vi "Acqusition & Generation (with Snapshot 3) test.vi"() -> ()   [LabVIEW 2014]
uses:
  <vilib>/Platform/TimedLoop/XDataNode/timing_clust.ctl
  <vilib>/Platform/TimedLoop/XDataNode/nitl_modes.ctl
  <vilib>/Platform/TimedLoop/XDataNode/wakeup.ctl
  <vilib>/rvi/Emulation/niFpgaSctlEmulationGetInTimedLoop.vi
  <vilib>/rvi/Emulation/niFpgaEmulationReportErrorSimple.vi
  <vilib>/rvi/Emulation/niFpgaGetClockAttributes.vi
  <vilib>/rvi/Emulation/niFpgaCriticalErrorInLSC.vi
  <vilib>/rvi/Emulation/niFpgaEmulationIsFPGAContextNoSignature.vi
  <vilib>/rvi/errors/niFpgaSetErrorForExecOnDevCompSimple.vi
  <vilib>/rvi/eio/common/nirviEmuReportErrorAndStop.vi
  <vilib>/rvi/DataTransferAndStorage/Container/Common/niFpgaContainerGetUniqueNameForEmu.vi
  <vilib>/rvi/FIFO/Fifo_Resource/nirvififoEmulationSetSize.vi
  <vilib>/rvi/FIFO/Fifo_Resource/nirviFifoEmulationQueueMgr.vi
  <instcachedir>/0/nirviFifoEmulationQueueMgr_E5CAEC123FF24DC58D834DCA3CDAA9B5.lvgen/nirviFifoEmulationQueueMgr_E5CAEC123FF24DC58D834DCA3CDAA9B5_010.vi
  <vilib>/rvi/FIFO/Fifo_Resource/nirvififoEmulationDetermineInputValidOut.vi
  <vilib>/rvi/FIFO/Fifo_Resource/nirvififoEmulationCreateLock.vi
  <vilib>/rvi/Emulation/niFpgaProcessEmulError.vi
  <vilib>/rvi/FIFO/Fifo_Resource/nirvififoEmulationObtainLock.vi
  <vilib>/rvi/FIFO/Fifo_Resource/nirvififoEmulationReleaseLock.vi
  <vilib>/rvi/occurrence/nirviWaitOnOccurrenceBase.vi
  <vilib>/rvi/errors/nirviReportUnexpectedCaseInternalError.vi
  <vilib>/rvi/errors/nirviReportUnexpectedCaseInternalError (U32).vi
  <vilib>/rvi/Memory/Memory_Emulation/nirvimemoryFastEmulation.vi
  <vilib>/rvi/Memory/Memory_Emulation/nirvimemoryEmulation.vi
  <vilib>/rvi/interface/RandomDataEmulation/niFpgaRandomDataHandleErrors.vi
  <vilib>/rvi/eio/common/nirviEmuTemplateMethod_errors.vi
  <vilib>/Platform/TimedLoop/XDataNode/XDataNode.xnode
  <vilib>/rvi/DataTransferAndStorage/Container/XNode/niFpgaContainer.xnode
  <vilib>/rvi/FIFO/Fifo_Resource/nirvififoEmulationWrite.vi
  <vilib>/rvi/interface/RandomDataEmulation/nirviRandomDataFpgaReadWriteTemplate.vi
  <vilib>/rvi/FIFO/Fifo_Resource/nirvififoEmulationRead.vi
  <vilib>/eio/EIOMethodNode/EIOMethodNode.xnode
  <vilib>/Platform/TimedLoop/XDataNode/XDNodeRunTimeDep.lvlib
panel:
  in  "Snapshot":bool
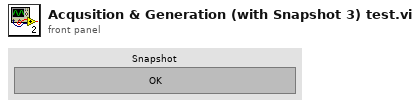
[diagram p1: front panel]
types:
  T1 = typedef "XDNodeRunTimeDep.lvlib/timing_clust.ctl" = cluster{"Expected End [f-1]":u64, "Actual End [f-1]":u64, "Finished Late? [f-1]":bool, "Expected End [i-1]":u64, "Actual End [i-1]":u64, "Finished Late? [i-1]":bool, "Expected Start [i]":u64, "Actual Start [i]":u64, "Expected Start [f]":u64, "Actual Start [f]":u64, "Source Name":string, "Structure Name":string, "Period":i64, "Deadline":i64, "Offset":i64, "Start":i64, "Priority":i32, "Timeout":i32, "Mode":T2, "Wakeup Reason":T3, "Error":errorcluster, "Source Type":string, "Secondary Source Type":string, "Global End Time":u64, "Global Start Time":u64, "Frame Duration":u64, "Iteration Duration":u64, "Assigned CPU":i32, "I/O Scan Engine Mode":u32}
  T2 = typedef "XDNodeRunTimeDep.lvlib/nitl_modes.ctl" = enum32{"No Change", "Process missed periods, maintain original phase", "Discard missed periods, maintain original phase", "Process missed periods, ignore original phase", "Discard missed periods, ignore original phase"}
  T3 = typedef "XDNodeRunTimeDep.lvlib/wakeup.ctl" = enum32{"Normal", "Aborted", "Asynchronous wakeup", "Timing source error", "Timed loop error", "Timeout"}
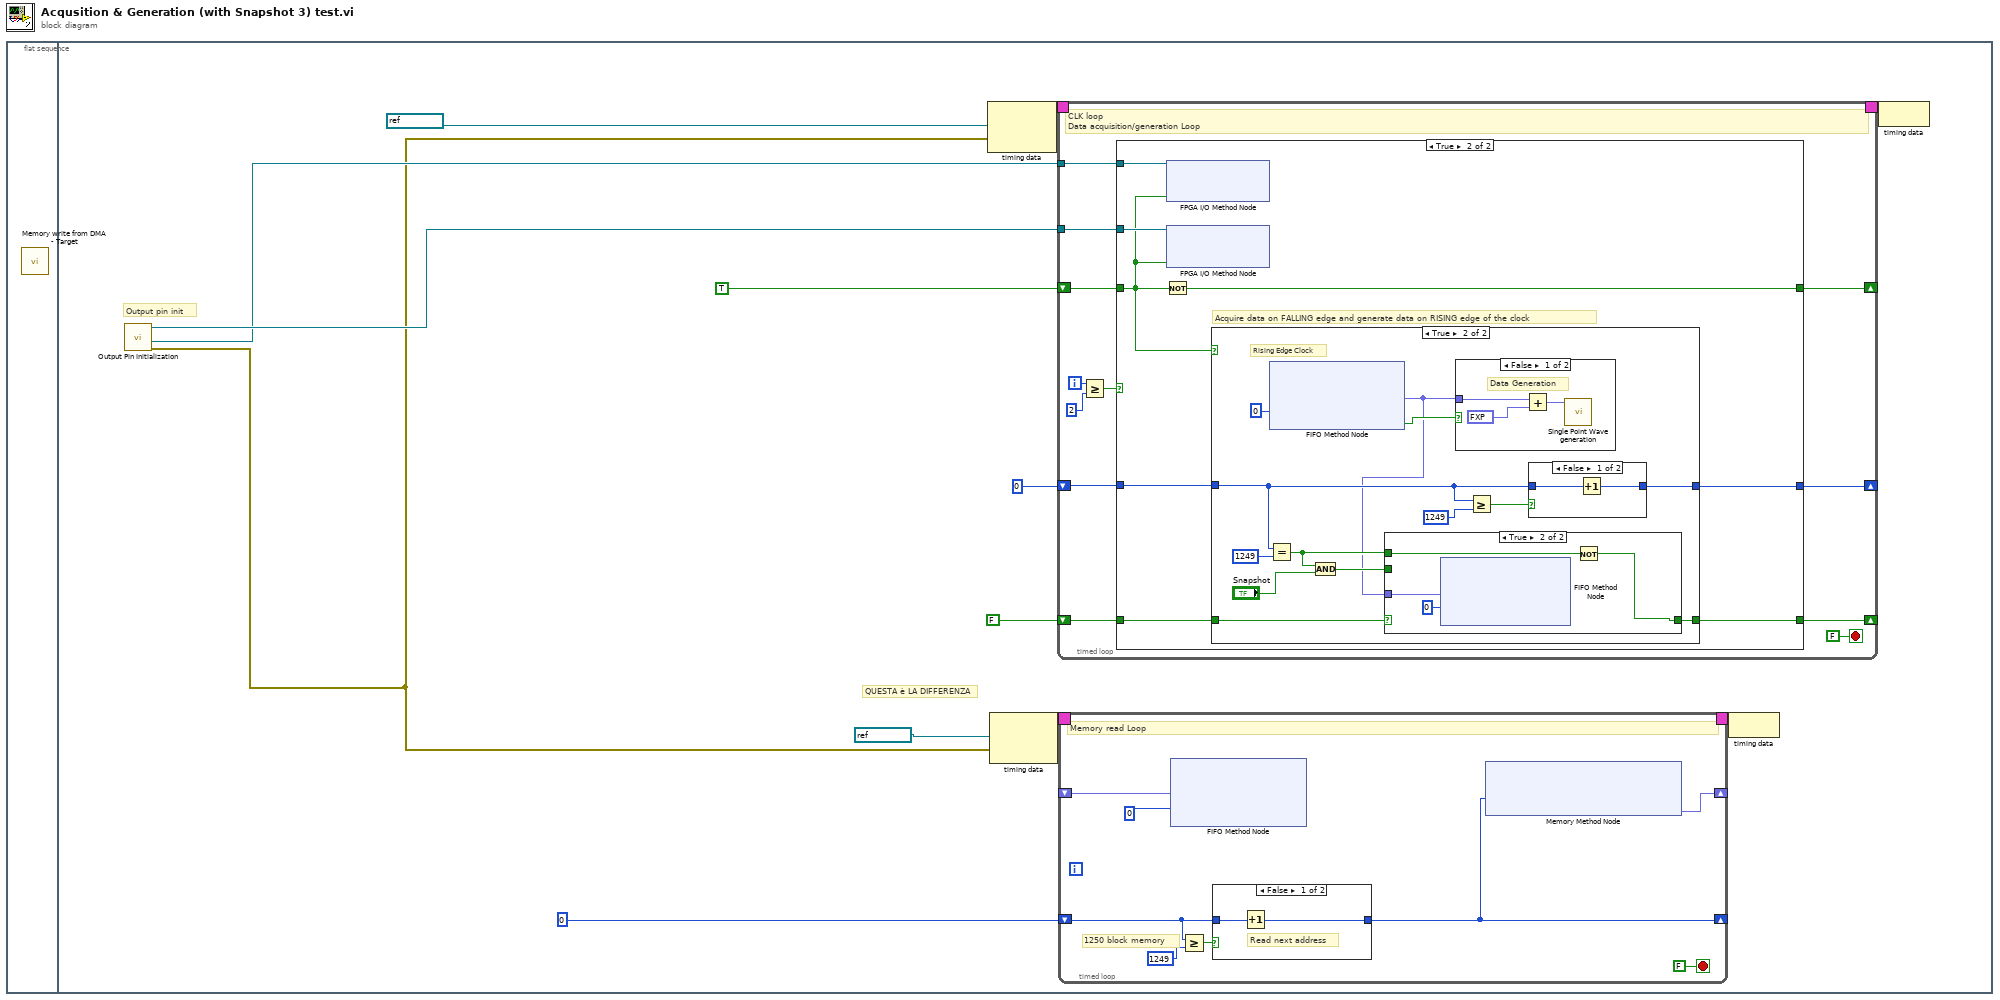
[diagram p0: block diagram]
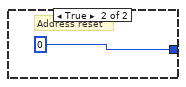
[diagram p2: hidden frame]
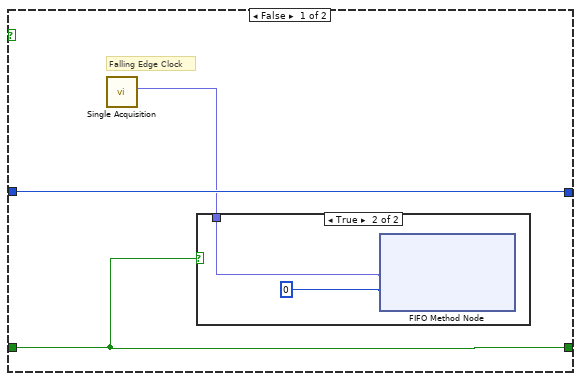
[diagram p4: hidden frame]
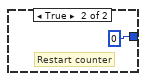
[diagram p8: hidden frame]
diagram:
  n1 = flat-sequence {
    frame #0 {
      n2 = call "Memory write from DMA - Target.vi"() -> ()  [unwired: 12 in]
    }
    frame #1 {
      # "QUESTA è LA DIFFERENZA"
      # "Output pin init"
      n3 = call "Output Pin Initialization.vi"() -> ("error out"=w3:errorcluster, "I/O Out Clock DAC (pin16)"=w4:refnum<k21>, "I/O Out Clock ADC (pin17)"=w5:refnum<k21>)  [unwired: 8 in]
      n4 = node-c288(refnum<k21> "100MHz" ("Source Name"), w3) -> (w13:T1)
      n5 = node-c288(refnum<k21> "100MHz" ("Source Name"), w3) -> (w11:T1)
      n6 = timed-loop {
        timing: w13 -> [_]
        timing-out: [_] -> w12
        shift-right: [w41] -> _
        shift-left: TRUE -> [w39]
        tunnel: w4 -> [w43]
        tunnel: w5 -> [w40]
        shift-right: [w38] -> _
        shift-left: i16 0 -> [w37]
        shift-right: [w35] -> _
        shift-left: FALSE -> [w36]
        i -> [w34]
        stop <- FALSE stop-if-true
        # "CLK loop\nData acquisition/generation Loop"
        n7 = Greater Or Equal?(x=w34, y=2) -> (x >= y?=w32:bool)
        n8 = case shown="True" w32 {
          tunnel: w43 -> [_ w54]
          tunnel: [w46 w53] -> w41
          tunnel: w40 -> [_ w52]
          tunnel: w39 -> [w46 w51]
          tunnel: [w45 w50] -> w38
          tunnel: w37 -> [w45 w49]
          tunnel: w36 -> [w44 w48]
          tunnel: [w44 w47] -> w35
          frame False {
          }
          frame True {
            # "Acquire data on FALLING edge and generate data on RISING edge of the clock"
            n9 = Not(x=w51) -> (.not. x?=w53:bool)
            n10 = xnode "FPGA I/O Method Node"("FPGA I/O In"=w54, "Data"=w51) -> ()  [unwired: 1 out]
            n11 = xnode "FPGA I/O Method Node"("FPGA I/O In"=w52, "Data"=w51) -> ()  [unwired: 1 out]
            n12 = case shown="True" w51 {
              tunnel: [w57 w70] -> w50
              tunnel: w49 -> [w57 w64]
              tunnel: w48 -> [w56 w67]
              tunnel: [w56 w65] -> w47
              frame False {
                # "Falling Edge Clock"
                n13 = call "Single Acquisition.vi"() -> ("Out"=w55:fxp<+/-,12,12>)  [unwired: 10 in, 1 out]
                n14 = case shown="True" w56 {
                  tunnel: w55 -> [_ w59]
                  frame False {
                  }
                  frame True {
                    n15 = xnode ("FIFO Method Node")("Element"=w59, "Timeout"=0) -> ()  [unwired: 1 in, 2 out]
                  }
                }
              }
              frame True {
                # "Rising Edge Clock"
                n16 = Equal?(x=w64, y=i16 1249) -> (x = y?=w63:bool)
                n17 = xnode ("FIFO Method Node")("Timeout"=0) -> ("Element"=w60:fxp<+/-,12,12>, "Timed Out?"=w61:bool)  [unwired: 1 in, 1 out]
                n18 = And(x=w63, y="Snapshot") -> (x .and. y?=w66:bool)
                n19 = case shown="True" w67 {
                  tunnel: w66 -> [w76 _]
                  tunnel: [w76 w79] -> w65
                  tunnel: w63 -> [_ w80]
                  tunnel: w60 -> [_ w78]
                  frame False {
                  }
                  frame True {
                    n20 = xnode ("FIFO Method Node")("Element"=w78, "Timeout"=0) -> ()  [unwired: 1 in, 2 out]
                    n21 = Not(x=w80) -> (.not. x?=w79:bool)
                  }
                }
                n22 = case shown="False" w61 {
                  tunnel: w60 -> [w75 _]
                  frame False {
                    # "Data Generation"
                    n23 = Add(x=w75, y=fxp<+,12,12> 2048.0) -> (x+y=w73:fxp<+/-,14,14>)
                    n24 = call "Single Point Wave generation.vi"("Data To Write"=w73) -> ()  [unwired: 10 in, 1 out]
                  }
                  frame True {
                    # "FPGA memory slow"
                  }
                }
                n25 = Greater Or Equal?(x=w64, y=i16 1249) -> (x >= y?=w71:bool)
                n26 = case shown="False" w71 {
                  tunnel: w64 -> [w82 _]
                  tunnel: [w81 i16 0] -> w70
                  frame False {
                    n27 = Increment(x=w82) -> (x+1=w81:i16)
                  }
                  frame True {
                    # "Restart counter"
                  }
                }
              }
            }
          }
        }
      }
      n28 = timed-loop {
        timing: w11 -> [_]
        timing-out: [_] -> w10
        shift-right: [w14] -> _
        shift-left: u32 0 -> [w18]
        shift-right: [w16] -> _
        shift-left: _ -> [w15]
        stop <- FALSE stop-if-true
        # "1250 block memory"
        # "Memory read Loop"
        n29 = xnode ("FIFO Method Node")("Element"=w15, "Timeout"=0) -> ()  [unwired: 1 in, 2 out]
        n30 = Greater Or Equal?(x=w18, y=u32 1249) -> (x >= y?=w20:bool)
        n31 = case shown="False" w20 {
          tunnel: w18 -> [w23 _]
          tunnel: [w22 u32 0] -> w14
          frame False {
            # "Read next address"
            n32 = Increment(x=w23) -> (x+1=w22:u32)
          }
          frame True {
            # "Address reset"
          }
        }
        n33 = xnode ("Memory Method Node")("Address"=w14) -> ("Data"=w16:fxp<+/-,12,12>)  [unwired: 1 in, 1 out]
      }
      n34 = node-c288(w10) -> ()
      n35 = node-c288(w12) -> ()
    }
  }
